vi "freqToStringvi.vi"(8 "error in (no error)":errorcluster, 11 "rf in":refnum<class "rf.lvclass">) -> (0 "error out":errorcluster, 2 "frequency":string, 3 "rf out":refnum<class "rf.lvclass">)   [LabVIEW 2009, in "Tools.lvlib" / "Scripting.lvlib" / "rf.lvclass"]
uses:
  rf.lvclass
  rf.lvclass/rf.ctl
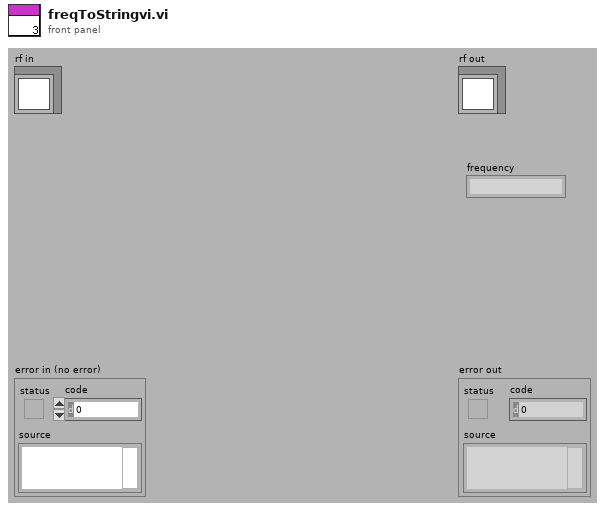
[diagram p1: front panel]
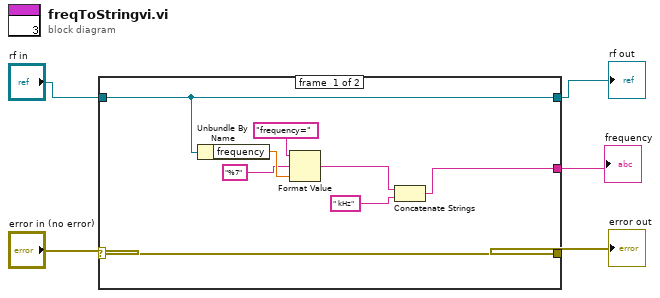
[diagram p0: block diagram]
diagram:
  n1 = case shown="No Error" "error in (no error)" {
    selector: "error in (no error)" -> [w11 w14]
    tunnel: [w11 w14] -> w4
    tunnel: [w10 w15] -> w2
    tunnel: "rf in" -> [w10 w15]
    tunnel: [w6 _] -> w1
    frame #0 {
      n2 = Unbundle By Name(w10) -> ("frequency"=w13:dbl)
      n3 = Format Value(string ("")="frequency=", format string="%7", value (0)=w13) -> (output string=w7:string)
      n4 = Concatenate Strings(w7, " kHz") -> (w6:string)
    }
    frame #1 {
    }
  }
  "error out" <- w4
  "rf out" <- w2
  "frequency" <- w1
